vi "Sort 2D Array.vi"   [LabVIEW 2025]
doc: "This polymorphic VI sorts a 2D array of numerics or strings, regardless of the array size. You can specify whether to sort by column or row, which column or row to sort by, and whether to sort in ascending or descending order. You also can specify a secondary row or column to sort by."
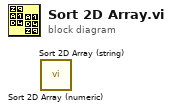
[diagram p0: block diagram]
diagram:
  n1 = call "Sort 2D Array (numeric).vi"() -> ()  [unwired: 5 in, 2 out]
  n2 = call "Sort 2D Array (string).vi"() -> ()  [unwired: 5 in, 2 out]
